vi "Read Discrete Inputs.vi"(8 "error in (no error)":errorcluster, 9 "number of inputs":u16, 10 "starting address":u16, 11 "device data model in":refnum<class "ICPCON ET Data Model.lvclass">) -> (0 "error out":errorcluster, 2 "data":bool[](array[boolean]), 3 "device data model out":refnum<class "ICPCON ET Data Model.lvclass">)   [LabVIEW 2021, in "ICPCON ET Data Model.lvclass"]
doc: "Reads N discrete inputs from the data model starting at address M."
uses:
  ICPCON ET Data Model.lvclass
  ICPCON ET Data Model.lvclass/ICPCON ET Data Model.ctl
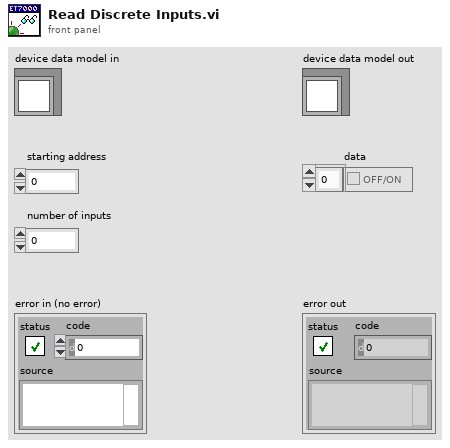
[diagram p1: front panel]
types:
  T1 = typedef "SubVIs.lvlib/ICPCON ET Data Model.lvclass/Data Model.ctl" = cluster{"UTC":u64, "DI":bool[], "DO":bool[], "IR":u16[], "HR":u16[], "ES":u8}
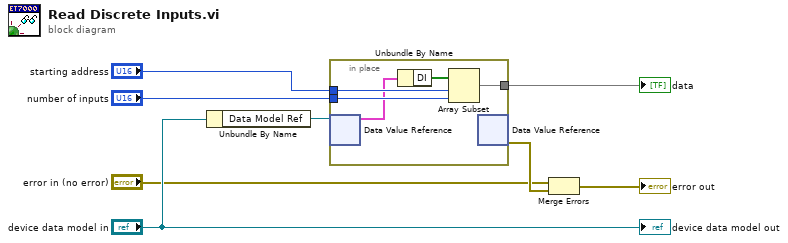
[diagram p0: block diagram]
diagram:
  n1 = Unbundle By Name("device data model in") -> ("Data Model Ref"=w3:refnum<data-value>)
  n2 = in-place {
    in-place-border: "starting address" -> [w13]
    in-place-border: "number of inputs" -> [w12]
    in-place-border: [w11] -> w4
    n3 = in-place-dvr #1(w3) -> (w10:T1)  [unwired: 1 out]
    n4 = Unbundle By Name(w10) -> ("DI"=w9:bool[])
    n5 = Array Subset(array=w9, index=w13, length=w12) -> (w11:bool[])
    n6 = in-place-dvr #1() -> (w2:errorcluster)  [unwired: 1 in, 1 out]
  }
  "data" <- w4
  n7 = Merge Errors("error in (no error)", w2) -> (→"error out":errorcluster)
  "device data model out" <- "device data model in"
